vi "FTW-Supervisor-CloseConnection.vi"(0 "FTW Supervisor Connection":refnum<class "FTW-Supervisor-Connector.lvclass">, 11 "error in":errorcluster) -> (15 "error out":errorcluster)   [LabVIEW 2014, in "FTW-Supervisor-Connector.lvclass"]
uses:
  FTW-Supervisor-Connector.lvclass
panel:
  # "Inputs"
  # "Outputs"
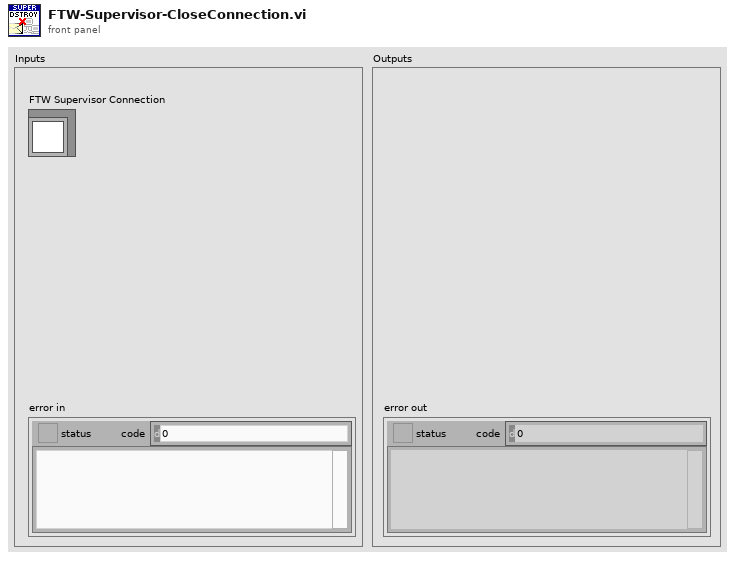
[diagram p1: front panel]
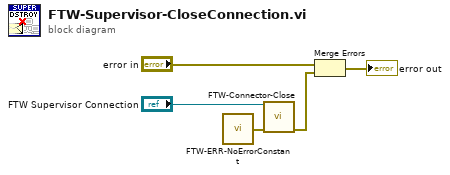
[diagram p0: block diagram]
diagram:
  n1 = call "FTW-ERR-NoErrorConstant.vi"() -> ("no error"=w2:errorcluster)
  n2 = call-dynamic "FTW-Connector-Close.vi"("FTW Actor Connector"="FTW Supervisor Connection", "error in"=w2) -> ("error out"=w1:errorcluster)  [unwired: 13 in]
  n3 = Merge Errors("error in", w1) -> (→"error out":errorcluster)
